vi "combined.vi"() -> ()   [LabVIEW 2020]
panel:
  out "Weed Status":string
  out "Scan Status":string
  out "Location Status":string
  in  "OK":bool
  in  "stop":bool
  in  "Start":bool
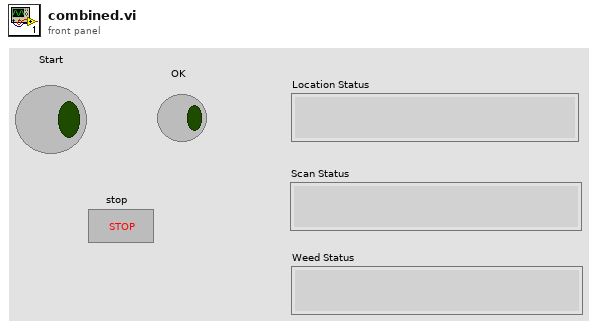
[diagram p1: front panel]
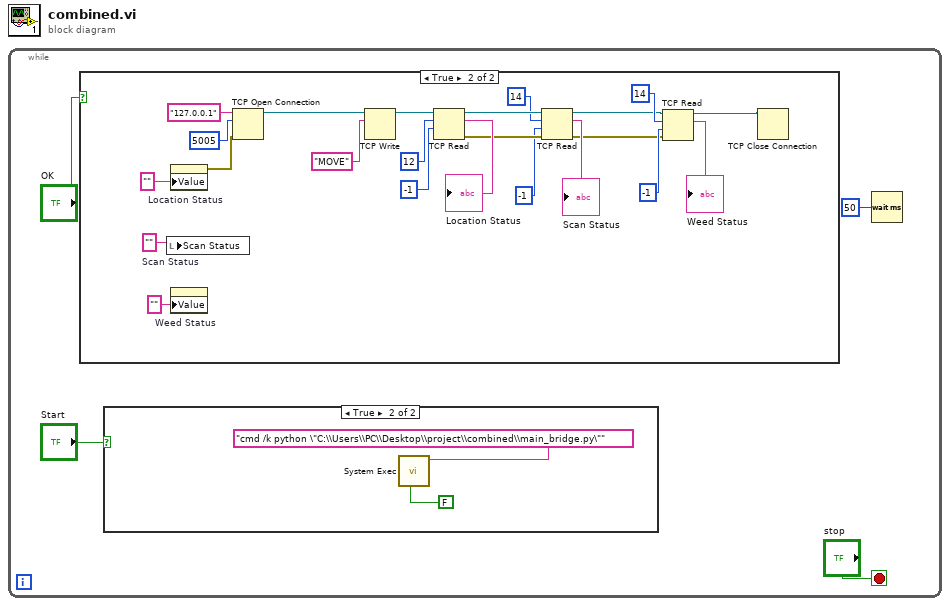
[diagram p0: block diagram]
diagram:
  n1 = while {
    stop <- "stop" stop-if-true
    n2 = case shown="True" "OK" {
      frame False {
      }
      frame True {
        w15 = ""  # Scan Status
        n3 = local write "Scan Status"(w15) -> ()
        n4 = property on="Location Status" class="Str"("Value"="" ("data out")) -> (error out=w20:errorcluster)  [unwired: 2 in, 1 out]
        n5 = property on="Weed Status" class="Str"("Value"="" ("Weed Status")) -> ()  [unwired: 2 in, 2 out]
        n6 = TCP Open Connection(address="127.0.0.1", remote port or service name=u16 5005, error in (no error)=w20) -> (connection ID=w27:refnum<k5>)  [unwired: 2 in, 1 out]
        n7 = TCP Write(connection ID=w27, data in="MOVE") -> (connection ID out=w25:refnum<k5>)  [unwired: 2 in, 2 out]
        n8 = TCP Read(connection ID=w25, bytes to read=12, 9:-1 ("timeout ms (25000)")) -> (connection ID out=w19:refnum<k5>, data out=→"Location Status":string, error out=w18:errorcluster)  [unwired: 2 in]
        n9 = TCP Read(connection ID=w19, bytes to read=14, error in (no error)=w18, 9:-1 ("timeout ms (25000)")) -> (connection ID out=w10:refnum<k5>, data out=→"Scan Status":string, error out=w9:errorcluster)  [unwired: 1 in]
        n10 = TCP Read(connection ID=w10, bytes to read=14, error in (no error)=w9, 9:-1 ("timeout ms (25000)")) -> (connection ID out=w8:refnum<k5>, data out=→"Weed Status":string)  [unwired: 1 in, 1 out]
        n11 = TCP Close Connection(connection ID=w8) -> ()  [unwired: 2 in, 2 out]
      }
    }
    n12 = case shown="True" "Start" {
      frame False {
      }
      frame True {
        n13 = call <vilib>:"System Exec.vi"("wait until completion? (T)"=FALSE, "command line"="cmd /k python \"C:\\Users\\PC\\Desktop\\project\\combined\\main_bridge.py\"") -> ()  [unwired: 6 in, 4 out]
      }
    }
    n14 = Wait (ms)(milliseconds to wait=u32 50) -> ()  [unwired: 1 out]
  }
